vi "step_set_hipot_I_limit.vi"(8 "error in":errorcluster, 10 "step":T3 {"data num" format="%.3f"}) -> (0 "error out":errorcluster, 2 "test results":T1)   [LabVIEW 2020]
uses:
  controls/PROTO_stepV2.ctl
  controls/MPB_step_type.ctl
  controls/test results.ctl
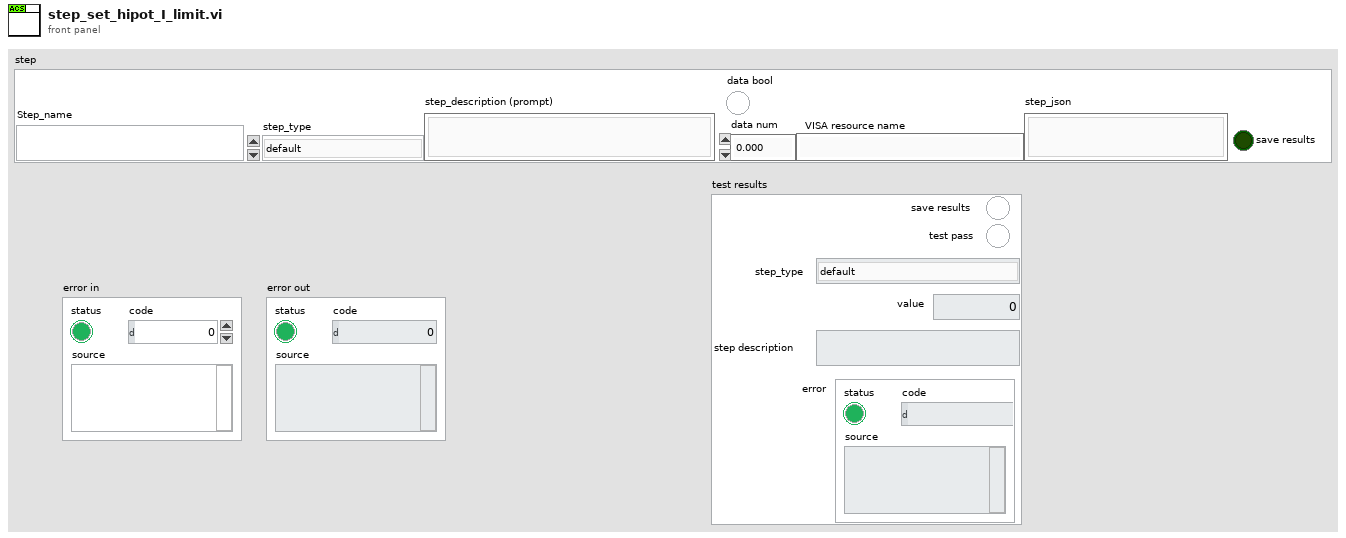
[diagram p1: front panel]
types:
  T1 = typedef "test results.ctl" = cluster{"test pass":bool, "step_type":T2, "value":dbl, "step description":string, "error":errorcluster, "save results":bool}
  T2 = typedef "MPB_step_type.ctl" = enum16{"default", "prompt", "sequence#", "12V_1_power supply on_off", "12V_2_power supply on_off", "set_hipot_V", "set_hipot_I_limit", "set_hipot_ramping (sec)", "set hipot_hold_time", "read_hipot_V", "read_hipot_I", "set_daq", "read_daq", "flash uds", "wait (sec)", "record_pass_fail", "ac_charge_test", "dc_400V_charging", "HAPS Heater Output", "HAPS Compressor Output", "stop_test", "error_exit"}
  T3 = typedef "PROTO_stepV2.ctl" = cluster{"VISA resource name":string, "data num":dbl, "step_description (prompt)":string, "step_json":string, "save results":bool, "step_type":T2, "Step_name":string, "data bool":bool}
  T4 = cluster{"error":bool, "code":i8, "source":string}
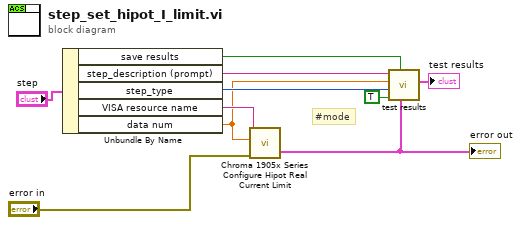
[diagram p0: block diagram]
diagram:
  # "#mode"
  n1 = Unbundle By Name("step") -> ("save results"=w1:bool, "step_description (prompt)"=w3:string, "step_type"=w5:T2, "VISA resource name"=w10:string, "data num"=w4:dbl)
  n2 = call <instrlib>:"Chroma 1905x Series Configure Hipot Real Current Limit.vi"("VISA session copy"=w10, "Real Current Limit"=w4, "error in"="error in") -> ("error out"=w6:T4)  [unwired: 2 in, 1 out]
  "error out" <- w6
  n3 = call "test results.vi"("error"=w6, "save results"=w1, "test pass"=TRUE, "step_type"=w5, "Numeric"=w4, "(description) used in test"=w3) -> ("test results"=→"test results":T1)  [unwired: 5 in]
